vi "XYZStage-Reset axis command.vi"(8 "error in (no error)":errorcluster, 9 "XYZ Stage dequeued data":T1={"Command"=enum."Initialize", "Channel"="Z", "X"=0.0, "Y"=0.0, "Z"=0.0, "Speed"=0, "Zero"=FALSE, "Use acknowledgement?"=TRUE} {"Speed" format="Speed= %.0f"; "Z" format="Z= %#_g"; "Y" format="Y= %#_g"; "X" format="X= %#_g"}, 10 "XY Stage":T4) -> (0 "error out":errorcluster)   [LabVIEW 2013]
uses:
  Typedefs/XY Stage config cluster.ctl
  Typedefs/XYZ stage data.ctl
  Typedefs/XYZ stage states.ctl
  Typedefs/XYZ channel ring.ctl
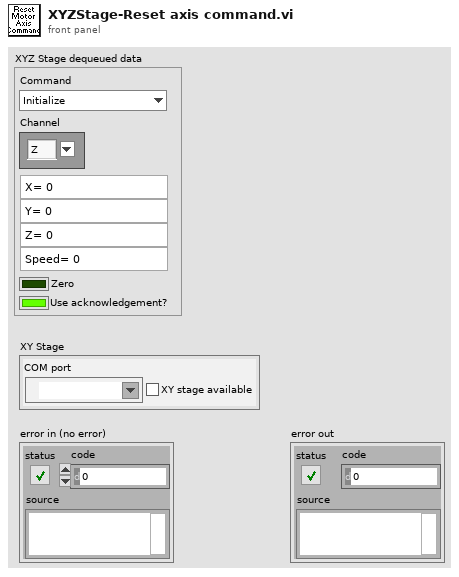
[diagram p1: front panel]
types:
  T1 = typedef "XYZ stage data.ctl" = cluster{"Command":T2, "Channel":T3, "X":sgl, "Y":sgl, "Z":sgl, "Speed":i32, "Zero":bool, "Use acknowledgement?":bool}
  T2 = typedef "XYZ stage states.ctl" = enum16{"Dequeue", "Initialize", "Read Position", "Read Speed Setting", "Move", "Set Max Speed", "Reset Axis", "Stop all movement"}
  T3 = typedef "XYZ channel ring.ctl" = string
  T4 = typedef "XY Stage config cluster.ctl" = cluster{"COM port":refnum<visa-resource-name>, "XY stage available":bool}
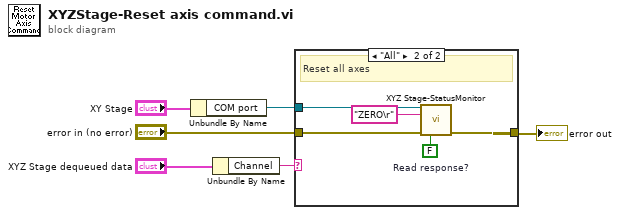
[diagram p0: block diagram]
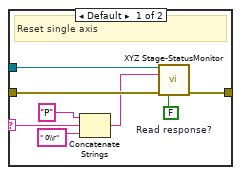
[diagram p2: hidden frame]
diagram:
  n1 = Unbundle By Name("XY Stage") -> ("COM port"=w1:refnum<visa-resource-name>)
  n2 = Unbundle By Name("XYZ Stage dequeued data") -> ("Channel"=w4:T3)
  n3 = case shown="\"All\"" w4 {
    selector: w4 -> [w10 _]
    tunnel: "error in (no error)" -> [w14 w19]
    tunnel: [w9 w18] -> w6
    tunnel: w1 -> [w8 w16]
    frame Default {
      w7 = FALSE  # Read response?
      # "Reset single axis"
      n4 = Concatenate Strings("P" ("string to write"), w10, " 0\\r" ("string")) -> (w11:string)
      n5 = call "XYZ Stage-StatusMonitor.vi"("VISA resource name"=w8, "string to write"=w11, "Error In"=w14, "Read response? (T)"=w7) -> ("Error Out"=w9:errorcluster)  [unwired: 7 in, 4 out]
    }
    frame "All" {
      w15 = FALSE  # Read response?
      # "Reset all axes"
      n6 = call "XYZ Stage-StatusMonitor.vi"("VISA resource name"=w16, "string to write"="ZERO\r", "Error In"=w19, "Read response? (T)"=w15) -> ("Error Out"=w18:errorcluster)  [unwired: 7 in, 4 out]
    }
  }
  "error out" <- w6
